vi "AxisCalc.vi"(5 "ScanAxis":T1, 6 "start":dbl, 8 "Number of pts\nper scan":i32, 9 "increment":dbl, 10 "Global Position (mm)":dbl[](array[numeric])) -> (3 "axis":T2)   [LabVIEW 2022 SP3]
uses:
  ScanningControl/Motion Controllers/-MotionRoutines/ScanAxis.ctl
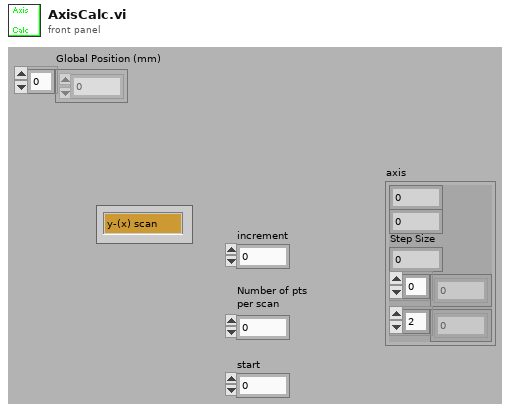
[diagram p1: front panel]
types:
  T1 = typedef "ScanAxis.ctl" = enum16{"y-(x) scan", "x-(y) scan", "z-(x) scan", "z-(y) scan", "y-(z) scan", "x-(z) scan", "w-(x) scan", "w-(y) scan", "w-(z) scan", "x-(w) scan", "y-(w) scan", "z-(w) scan"}
  T2 = cluster{"Axis 1 Start":dbl, "Axis 2 Start":dbl, "Step Size":dbl, "Axis 1 Ticks":dbl[], "Axis 2 Ticks":dbl[]}
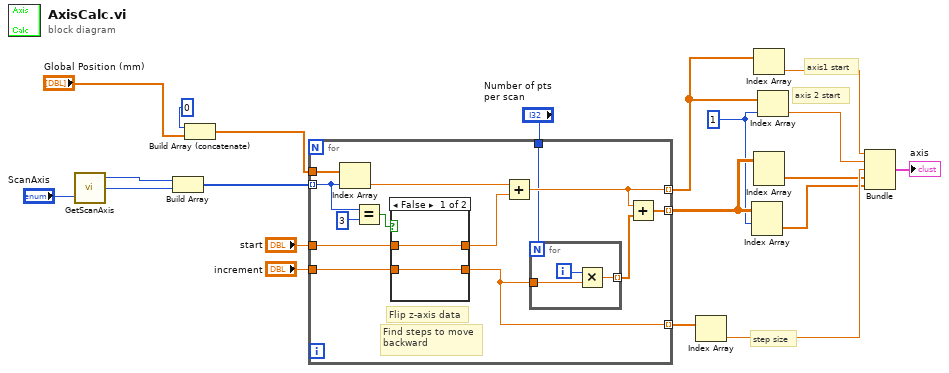
[diagram p0: block diagram]
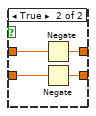
[diagram p2: hidden frame]
diagram:
  w9 = 1
  # "step size"
  # "axis 2 start"
  # "axis1 start"
  n1 = call "GetScanAxis.vi"("scan pair"="ScanAxis") -> ("Axis 1"=w5:i32, "Axis 2"=w4:i32)  [unwired: 1 in, 1 out]
  n2 = Build Array(w5, w4) -> (w17:i32[])
  n3 = Build Array (concatenate)(0, "Global Position (mm)") -> (w16:dbl[])
  n4 = for {
    tunnel: "increment" -> [w31]
    tunnel: "start" -> [w30]
    tunnel: w17 -> [w28] mode=indexing
    tunnel: w16 -> [w29]
    tunnel: [w24] -> w15 mode=indexing
    tunnel: [w23] -> w14 mode=indexing
    tunnel: [w22] -> w11 mode=indexing
    tunnel: "Number of pts\nper scan" -> [w21]
    # "Find steps to move\nbackward"
    # "Flip z-axis data"
    n5 = Index Array(array=w29, index=w28) -> (element=w27:dbl)
    n6 = Equal?(x=w28, y=3) -> (x = y?=w32:bool)
    n7 = case shown="False" w32 {
      tunnel: w31 -> [w35 w39]
      tunnel: w30 -> [w34 w38]
      tunnel: [w35 w37] -> w22
      tunnel: [w34 w36] -> w26
      frame False {
      }
      frame True {
        n8 = Negate(x=w38) -> (-x=w36:dbl)
        n9 = Negate(x=w39) -> (-x=w37:dbl)
      }
    }
    n10 = Add(x=w27, y=w26) -> (x+y=w24:dbl)
    n11 = for {
      N: w21 -> [_]
      tunnel: w22 -> [w41]
      tunnel: [w40] -> w25 mode=indexing
      i -> [w42]
      n12 = Multiply(x=w42, y=w41) -> (x*y=w40:dbl)
    }
    n13 = Add(x=w24, y=w25) -> (x+y=w23:dbl[])
  }
  n14 = Index Array(array=w11) -> (element=w10:dbl)  [unwired: 1 in]
  n15 = Index Array(array=w14, index (row)=w9) -> (element=w2:dbl[])  [unwired: 1 in]
  n16 = Index Array(array=w15) -> (element=w13:dbl)  [unwired: 1 in]
  n17 = Index Array(array=w14) -> (element=w3:dbl[])  [unwired: 2 in]
  n18 = Index Array(array=w15, index=w9) -> (element=w12:dbl)
  n19 = Bundle(w13, w12, "increment"=w10, w3, w2) -> (→"axis":cluster{dbl, dbl, "increment":dbl, dbl[], dbl[]})  [unwired: 1 out]
